vi "Pid_v01.vi"() -> ()   [LabVIEW 2010]
panel:
  in  "stop":bool
  out "u,y,r":cluster{"y":dbl, "u":dbl, "r-Set point":dbl}(graph)={"y"=50.04611274315553, "u"=50.10510244223579, "r-Set point"=50.0}
  in  "Kd":dbl(slide)=0.1151685393258427 scale=0.0..0.5
  in  "Ki":dbl(slide)=0.8764044943820224 scale=0.0..2.0
  in  "Kp":dbl(slide)=0.33707865168539325 scale=0.0..2.5
  out "y-Iesirea":dbl(slide)=50.04611274315553 scale=40.0..60.0
  out "u-Comanda":dbl(slide)=50.10510244223579 scale=40.0..60.0
  in  "r-Set point":dbl(slide)=50.0 scale=40.0..60.0
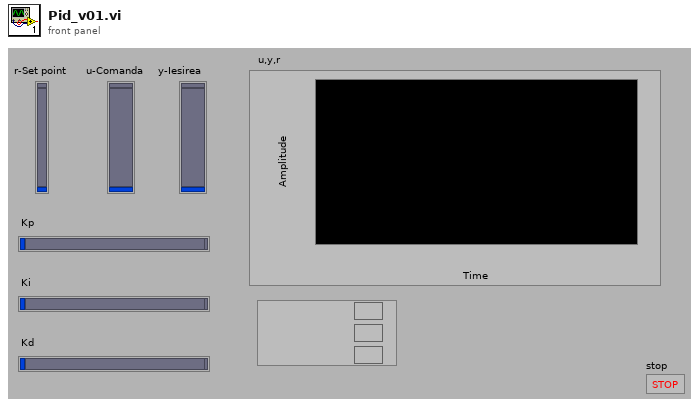
[diagram p1: front panel]
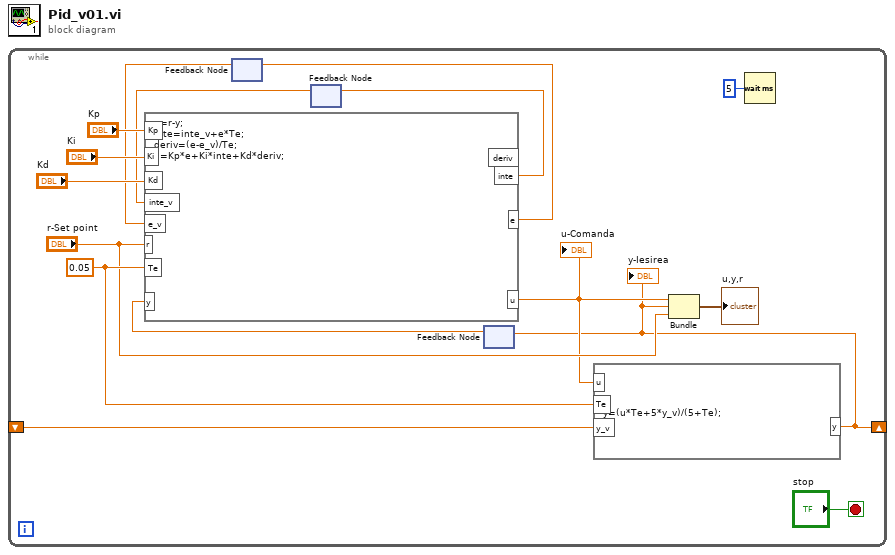
[diagram p0: block diagram]
diagram:
  n1 = while {
    shift-right: [w1] -> _
    shift-left: _ -> [w6]
    stop <- "stop" stop-if-true
    w5 = 0.05 ("input variable")
    n2 = feedback #1() -> (w10:dbl)  [unwired: 1 in]
    n3 = feedback #2() -> (w12:dbl)  [unwired: 1 in]
    n4 = feedback #3() -> (w7:dbl)  [unwired: 1 in]
    n5 = formula code="e=r-y;\ninte=inte_v+e*Te;\nderiv=(e-e_v)/Te;\nu=Kp*e+Ki*inte+Kd*deriv;"("Kp"="Kp", "Ki"="Ki", "Kd"="Kd", "inte_v"=w12, "e_v"=w10, "r"="r-Set point", "Te"=w5, "y"=w7) -> ("inte"=w13:dbl, "e"=w11:dbl, "u"=w3:dbl)  [unwired: 1 out]
    "u-Comanda" <- w3
    n6 = feedback-in #1(w11) -> ()
    n7 = feedback-in #2(w13) -> ()
    n8 = formula code="y=(u*Te+5*y_v)/(5+Te);"("u"=w3, "Te"=w5, "y_v"=w6) -> ("y"=w1:dbl)
    "y-Iesirea" <- w1
    n9 = feedback-in #3(w1) -> ()
    n10 = Bundle("u"=w3, "y"=w1, "r-Set point"="r-Set point") -> (→"u,y,r":cluster{"u":dbl, "y":dbl, "r-Set point":dbl})  [unwired: 1 in]
    n11 = Wait (ms)(milliseconds to wait=u32 5) -> ()  [unwired: 1 out]
  }
